vi "PH_Beckhoff.concatenate Klemmenstrings.vi"(3 "# of In- or Outputs":i32, 4 "Type":enum16{"AE", "AA", "DE", "DA", "SE"}(ring), 5 "Klemmenname":string, 6 "Quantity":i32) -> (0 "concatenated string array":string[](array[string]), 1 "\"and <Quantity> x <Klemmenname>\"":string, 2 "\"<Type>: <Quantity> x <Klemmenname>\"":string)   [LabVIEW 2014, in "PH_Beckhoff.lvlib"]
doc: "This VI creates a string array of this form:\n\n \"<Type>: [1 ... Quantitiy].<Klemmenname>.[1 ... #] - \""
uses:
  PH_Beckhoff.lvlib
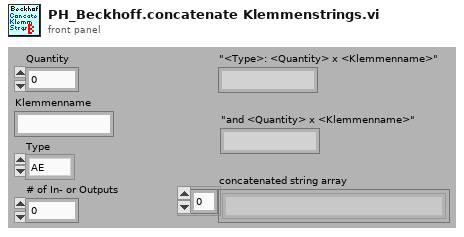
[diagram p1: front panel]
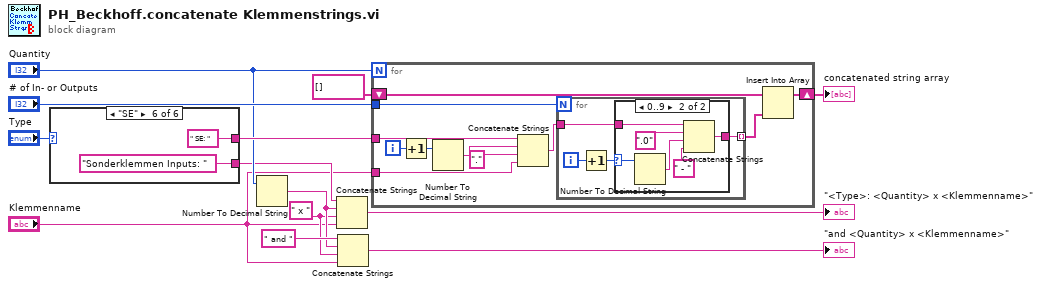
[diagram p0: block diagram]
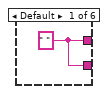
[diagram p2: hidden frame]
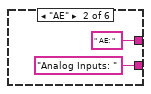
[diagram p3: hidden frame]
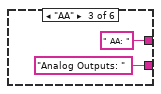
[diagram p4: hidden frame]
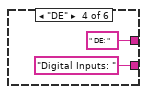
[diagram p5: hidden frame]
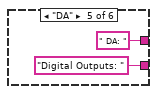
[diagram p6: hidden frame]
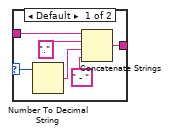
[diagram p7: hidden frame]
diagram:
  w3 = " x " ("string")
  n1 = case shown="\"SE\"" "Type" {
    tunnel: [w14 " AE: " " AA: " " DE: " " DA: " " SE: "] -> w9
    tunnel: [w14 "Analog Inputs: " "Analog Outputs: " "Digital Inputs: " "Digital Outputs: " "Sonderklemmen Inputs: "] -> w6
    frame Default {
      w14 = " "
    }
    frame "AE" {
    }
    frame "AA" {
    }
    frame "DE" {
    }
    frame "DA" {
    }
    frame "SE" {
    }
  }
  n2 = Number To Decimal String(number="Quantity") -> (decimal integer string=w4:string)  [unwired: 1 in]
  n3 = Concatenate Strings(w6, w4, w3, "Klemmenname") -> (→"\"<Type>: <Quantity> x <Klemmenname>\"":string)
  n4 = Concatenate Strings(" and " ("string"), w4, w3, "Klemmenname") -> (→"\"and <Quantity> x <Klemmenname>\"":string)
  n5 = for {
    N: "Quantity" -> [_]
    shift-right: [w35] -> w13
    shift-left: string[] [] -> [w33]
    tunnel: "Klemmenname" -> [w25]
    tunnel: "# of In- or Outputs" -> [w27]
    tunnel: w9 -> [w26]
    i -> [w32]
    n6 = Increment(x=w32) -> (x+1=w31:i32)
    n7 = Number To Decimal String(number=w31) -> (decimal integer string=w30:string)  [unwired: 1 in]
    n8 = Concatenate Strings(w26, w30, "." ("string"), w25) -> (w29:string)
    n9 = for {
      N: w27 -> [_]
      tunnel: [w38] -> w34 mode=indexing
      tunnel: w29 -> [w39]
      i -> [w37]
      n10 = Increment(x=w37) -> (x+1=w36:i32)
      n11 = case shown="0..9" w36 {
        selector: w36 -> [w40 w46]
        tunnel: w39 -> [w45 w51]
        tunnel: [w41 w47] -> w38
        frame Default {
          n12 = Number To Decimal String(number=w40) -> (decimal integer string=w43:string)  [unwired: 1 in]
          n13 = Concatenate Strings(w45, "." ("string"), w43, " - " ("string")) -> (w41:string)
        }
        frame 0..9 {
          n14 = Number To Decimal String(number=w46) -> (decimal integer string=w49:string)  [unwired: 1 in]
          n15 = Concatenate Strings(w51, ".0" ("string"), w49, " - " ("string")) -> (w47:string)
        }
      }
    }
    n16 = Insert Into Array(array=w33, new element=w34) -> (w35:string[])  [unwired: 1 in]
  }
  "concatenated string array" <- w13
